vi "PH_DataViewer.check GUI refs.vi"(0 "i ref in":refnum<vi>, 5 "error in (no error)":errorcluster) -> (14 "i ref out":refnum<vi>, 19 "error out":errorcluster)   [LabVIEW 2014, in "PH_DataViewer.lvlib"]
doc: "This Vi checks wether the GUI object references are valid."
uses:
  PH_DataViewer.lvlib
panel:
  out "Ref Timeout":bool
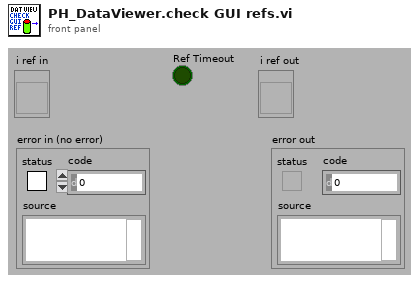
[diagram p1: front panel]
types:
  T1 = typedef "PH_DataViewer.lvlib/PH_DataViewer.i attribute.ctl" = cluster{"Images":cluster{"CAM":cluster{string, u32}, "BACKGROUND":cluster{string, u32}, "OPERATOR":cluster{string, u32}}, "Cam Operator GUI Refs":cluster{"Date Operators":refnum<vi>, "Time Operators":refnum<vi>, "Status Cali Data":refnum<vi>, "Calibration data":refnum<vi>, "Background Image":refnum<vi>, "Bg subtracted":refnum<vi>, "Op Image":refnum<vi>, "Cam Settings Operator":refnum<vi>, "Energy on":refnum<vi>, "exp Energy":refnum<vi>, "Energy":refnum<vi>, "Beam Analysis":refnum<vi>, "Analysis Type":refnum<vi>, "BA: Steps":refnum<vi>, "BA: Factor for ROI":refnum<vi>, "CoG - X":refnum<vi>, "CoG - Y":refnum<vi>, "Maj Diam":refnum<vi>, "Min Diam":refnum<vi>, "Phi":refnum<vi>, "Epsilon":refnum<vi>, "Phi rel to maj":refnum<vi>, "Position":refnum<vi>, "Position Type":refnum<vi>, "exp - X":refnum<vi>, "exp - Y":refnum<vi>, "Magni":refnum<vi>, "Foc Length":refnum<vi>, "Delta":refnum<vi>, "Theta":refnum<vi>, "Fit Gauss":refnum<vi>, "Maj Fit Order":refnum<vi>, "Min Fit Order":refnum<vi>, "Maj FWHM":refnum<vi>, "Min FWHM":refnum<vi>, "Maj 1 %":refnum<vi>, "Min 1 %":refnum<vi>}}
  T2 = cluster{"Date Operators":refnum<vi>, "Time Operators":refnum<vi>, "Status Cali Data":refnum<vi>, "Calibration data":refnum<vi>, "Background Image":refnum<vi>, "Bg subtracted":refnum<vi>, "Op Image":refnum<vi>, "Cam Settings Operator":refnum<vi>, "Energy on":refnum<vi>, "exp Energy":refnum<vi>, "Energy":refnum<vi>, "Beam Analysis":refnum<vi>, "Analysis Type":refnum<vi>, "BA: Steps":refnum<vi>, "BA: Factor for ROI":refnum<vi>, "CoG - X":refnum<vi>, "CoG - Y":refnum<vi>, "Maj Diam":refnum<vi>, "Min Diam":refnum<vi>, "Phi":refnum<vi>, "Epsilon":refnum<vi>, "Phi rel to maj":refnum<vi>, "Position":refnum<vi>, "Position Type":refnum<vi>, "exp - X":refnum<vi>, "exp - Y":refnum<vi>, "Magni":refnum<vi>, "Foc Length":refnum<vi>, "Delta":refnum<vi>, "Theta":refnum<vi>, "Fit Gauss":refnum<vi>, "Maj Fit Order":refnum<vi>, "Min Fit Order":refnum<vi>, "Maj FWHM":refnum<vi>, "Min FWHM":refnum<vi>, "Maj 1 %":refnum<vi>, "Min 1 %":refnum<vi>}
  T3 = cluster{"Date Operators":bool, "Time Operators":bool, "Status Cali Data":bool, "Calibration data":bool, "Background Image":bool, "Bg subtracted":bool, "Op Image":bool, "Cam Settings Operator":bool, "Energy on":bool, "exp Energy":bool, "Energy":bool, "Beam Analysis":bool, "Analysis Type":bool, "BA: Steps":bool, "BA: Factor for ROI":bool, "CoG - X":bool, "CoG - Y":bool, "Maj Diam":bool, "Min Diam":bool, "Phi":bool, "Epsilon":bool, "Phi rel to maj":bool, "Position":bool, "Position Type":bool, "exp - X":bool, "exp - Y":bool, "Magni":bool, "Foc Length":bool, "Delta":bool, "Theta":bool, "Fit Gauss":bool, "Maj Fit Order":bool, "Min Fit Order":bool, "Maj FWHM":bool, "Min FWHM":bool, "Maj 1 %":bool, "Min 1 %":bool}
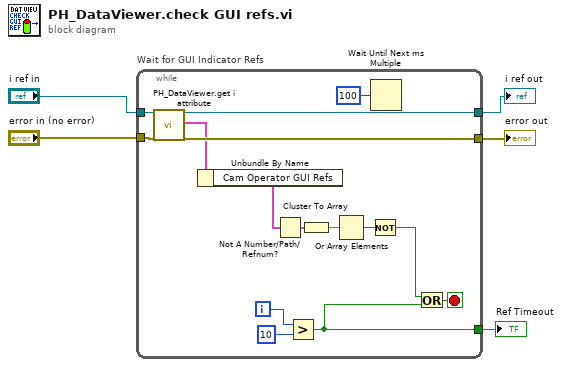
[diagram p0: block diagram]
diagram:
  n1 = while "Wait for GUI Indicator Refs" {
    tunnel: "i ref in" -> [w20]
    tunnel: "error in (no error)" -> [w19]
    tunnel: [w13] -> w3
    tunnel: [w15] -> w4
    tunnel: [w14] -> w5
    i -> [w17]
    stop <- w12 stop-if-true
    n2 = call "PH_DataViewer.get i attribute.vi"("i ref in"=w20, "error in (no error)"=w19) -> ("i ref out"=w15:refnum<vi>, "i attribute"=w11:T1, "error out"=w14:errorcluster)  [unwired: 15 in]
    n3 = Unbundle By Name(w11) -> ("Cam Operator GUI Refs"=w7:T2)
    n4 = Not A Number/Path/Refnum?(number/path/refnum=w7) -> (NaN/Path/Refnum?=w10:T3)
    n5 = Greater?(x=w17, y=10) -> (0:w13:bool)
    n6 = Cluster To Array(cluster=w10) -> (array=w9:bool[])
    n7 = Or Array Elements(Boolean array=w9) -> (logical OR=w8:bool)
    n8 = Not(x=w8) -> (.not. x?=w6:bool)
    n9 = Wait Until Next ms Multiple(millisecond multiple=u32 100) -> ()  [unwired: 1 out]
    n10 = Or(x=w6, y=w13) -> (x .or. y?=w12:bool)
  }
  "Ref Timeout" <- w3
  "error out" <- w5
  "i ref out" <- w4
